vi "Orca Flash Get Current Frame.vi"(0 "Camera Notifier Name":string) -> (4 "Camera Notifier Name (Dup)":string, 8 "Current Frame":u32)   [LabVIEW 2025]
uses:
  Camera Controls/Camera IMAQ Key Info.ctl
  Orca Flash Controls/Orca Flash Actions.ctl
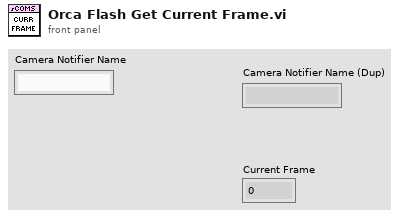
[diagram p1: front panel]
types:
  T1 = typedef "Orca Flash Actions.ctl" = enum16{"Idle", "Preview", "Record", "Record Settings", "Set Param", "Get Param", "Set ROI", "Get ROI", "Trigger Source", "Trigger Type", "Progessive Mode", "Area Mode", "Status", "Quit"}
  T2 = typedef "Camera IMAQ Key Info.ctl" = cluster{"Frame":u32, "Sensor Height":i32, "Sensor Width":i32, "ROI Height":i32, "ROI Width":i32, "ROI Enable?":bool, "Bit per Pixel":u8}
  T3 = typedef "IMAQ Image.ctl" = refnum<image>
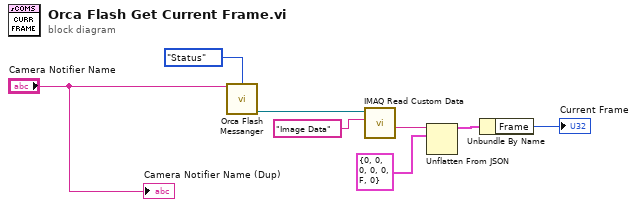
[diagram p0: block diagram]
diagram:
  n1 = call "Orca Flash Messanger.vi"("Notifier Name"="Camera Notifier Name", "Camera Actions"=Orca_Flash_Actions."Status") -> ("Image Ref"=w4:T3)  [unwired: 9 in, 4 out]
  n2 = call "IMAQ Read Custom Data"("Key"="Image Data", "Image"=w4) -> ("Custom Data Out"=w6:string)  [unwired: 7 in, 2 out]
  n3 = Unflatten From JSON(JSON string=w6, type and defaults=T2 {"Frame"=0, "Sensor Height"=0, "Sensor Width"=0, "ROI Height"=0, "ROI Width"=0, "ROI Enable?"=FALSE, "Bit per Pixel"=0} ("Camera IMAQ Key Info")) -> (value=w8:T2)  [unwired: 5 in, 1 out]
  n4 = Unbundle By Name(w8) -> ("Frame"=→"Current Frame":u32)
  "Camera Notifier Name (Dup)" <- "Camera Notifier Name"
